vi "get_current_read_position.vi"(8 "error in (no error)":errorcluster, 11 "DAQmxWriteSignals in":refnum<class "SignalWriterMM140725DAQmx.lvclass">) -> (0 "error out":errorcluster, 2 "current read position":dbl, 3 "DAQmxWriteSignals out":refnum<class "SignalWriterMM140725DAQmx.lvclass">)   [LabVIEW 2010, in "SignalWriterMM140725DAQmx.lvclass"]
uses:
  SignalWriterMM140725DAQmx.lvclass
  Program Files (x86)/National Instruments/LabVIEW 2010/resource/objmgr/daqmx.rc
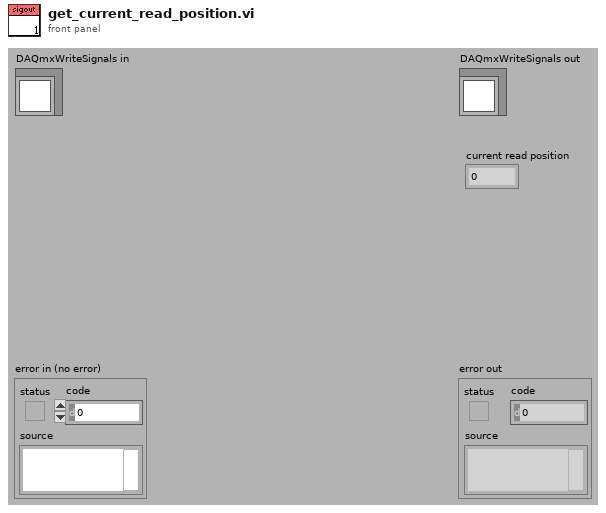
[diagram p1: front panel]
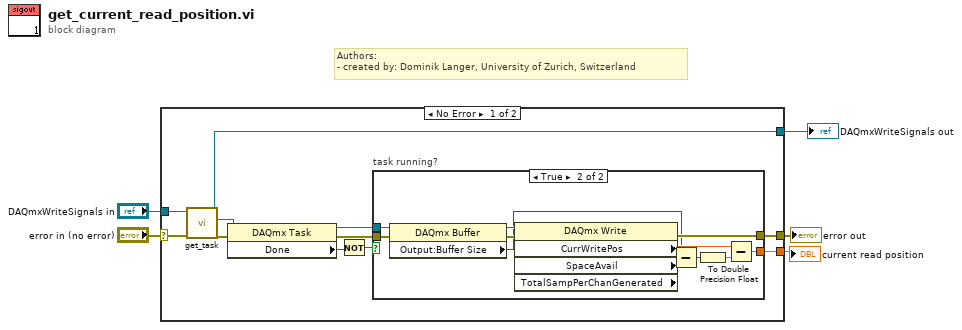
[diagram p0: block diagram]
diagram:
  # "Authors: \n- created by: Dominik Langer, University of Zurich, Switzerland"
  n1 = case shown="No Error" "error in (no error)" {
    selector: "error in (no error)" -> [w16 w30]
    tunnel: [w13 w30] -> w4
    tunnel: [w14 w29] -> w2
    tunnel: "DAQmxWriteSignals in" -> [w15 w29]
    tunnel: [w6 _] -> w1
    frame No Error {
      n2 = call-dynamic "get_task.vi"("error in (no error)"=w16, "DAQmxWriteSignals in"=w15) -> ("error out"=w12:errorcluster, "writer task"=w10:refnum<k21>, "DAQmxWriteSignals out"=w14:refnum<class "SignalWriterMM140725DAQmx.lvclass">)  [unwired: 7 out]
      n3 = property class="DAQmx Task"(reference=w10, error in=w12) -> (reference out=w9:refnum<k21>, error out=w11:errorcluster, "Done"=w8:bool)
      n4 = Not(x=w8) -> (.not. x?=w7:bool)
      n5 = case "task running?" shown="True" w7 {
        tunnel: [w17 w28] -> w13
        tunnel: w11 -> [w17 w25]
        tunnel: w9 -> [_ w24]
        tunnel: [_ w20] -> w6
        frame False {
        }
        frame True {
          n6 = property class="DAQmx Buffer"(reference=w24, error in=w25) -> (reference out=w22:refnum<k21>, error out=w23:errorcluster, "Output:Buffer Size"=w21:u32)
          n7 = property class="DAQmx Write" props=["CurrWritePos", "SpaceAvail", "TotalSampPerChanGenerated"](reference=w22, error in=w23) -> (error out=w28:errorcluster, "CurrWritePos"=w27:dbl, "SpaceAvail"=w26:u32)  [unwired: 2 out]
          n8 = Subtract(x=w21, y=w26) -> (x-y=w18:u32)
          n9 = To Double Precision Float(number=w18) -> (double precision float=w19:dbl)
          n10 = Subtract(x=w27, y=w19) -> (x-y=w20:dbl)
        }
      }
    }
    frame Error {
    }
  }
  "error out" <- w4
  "DAQmxWriteSignals out" <- w2
  "current read position" <- w1
